vi "Tester.vi"() -> ()   [LabVIEW 2015]
uses:
  controls/Treatment Parameters.ctl
  controls/Results.ctl
panel:
  out "adjust limbus time":u32
  out "sclera plane time":u32
  in  "Results folder":path=path "S:/Dropbox/clients/BELKIN/Results Small"
  in  "Treatment":T1={"Location"=25.0, "Width"=10.0, "Search"=enum."Lower"}
  out "error out":errorcluster
  in  "Image folder":path=path "S:/Dropbox/clients/BELKIN/Images and Requirements/BELKIN_-_Basler-2015-10-05/BELKIN - Basler/Representative Subset"
  out "Output Image":T2(plugin-control)
  out "Input Image":T2(plugin-control)
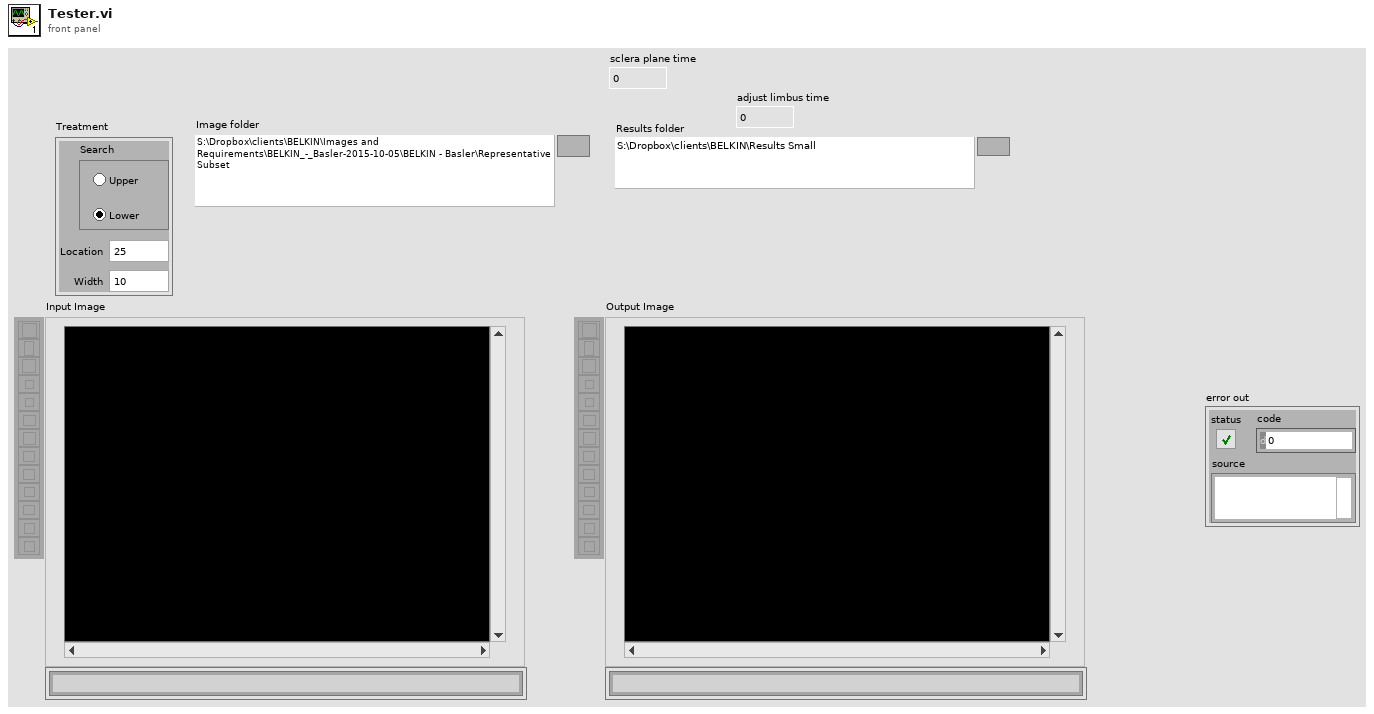
[diagram p1: front panel]
types:
  T1 = typedef "Treatment Parameters.ctl" = cluster{"Location":dbl, "Width":dbl, "Search":enum32{"Upper", "Lower"}}
  T2 = typedef "IMAQ Image.ctl" = refnum<image>
  T3 = typedef "Results.ctl" = cluster{"Center X":i32, "Center Y":i32, "Radius X":i32, "Radius Y":i32, "Circle Match Score":i32, "Sclera Score":dbl, "Circle Fit Strength":i32, "Circle Match Threshold":i32}
  T4 = typedef "Images.ctl" = cluster{"Input":T2, "Output":T2, "BufferGray1":T2, "BufferGray2":T2, "TemplatesDown":T2[], "TemplatesUp":T2[], "BufferColor1":T2, "GreenPlane":T2, "ScleraPlane":T2, "RedPlane":T2, "BluePlane":T2}
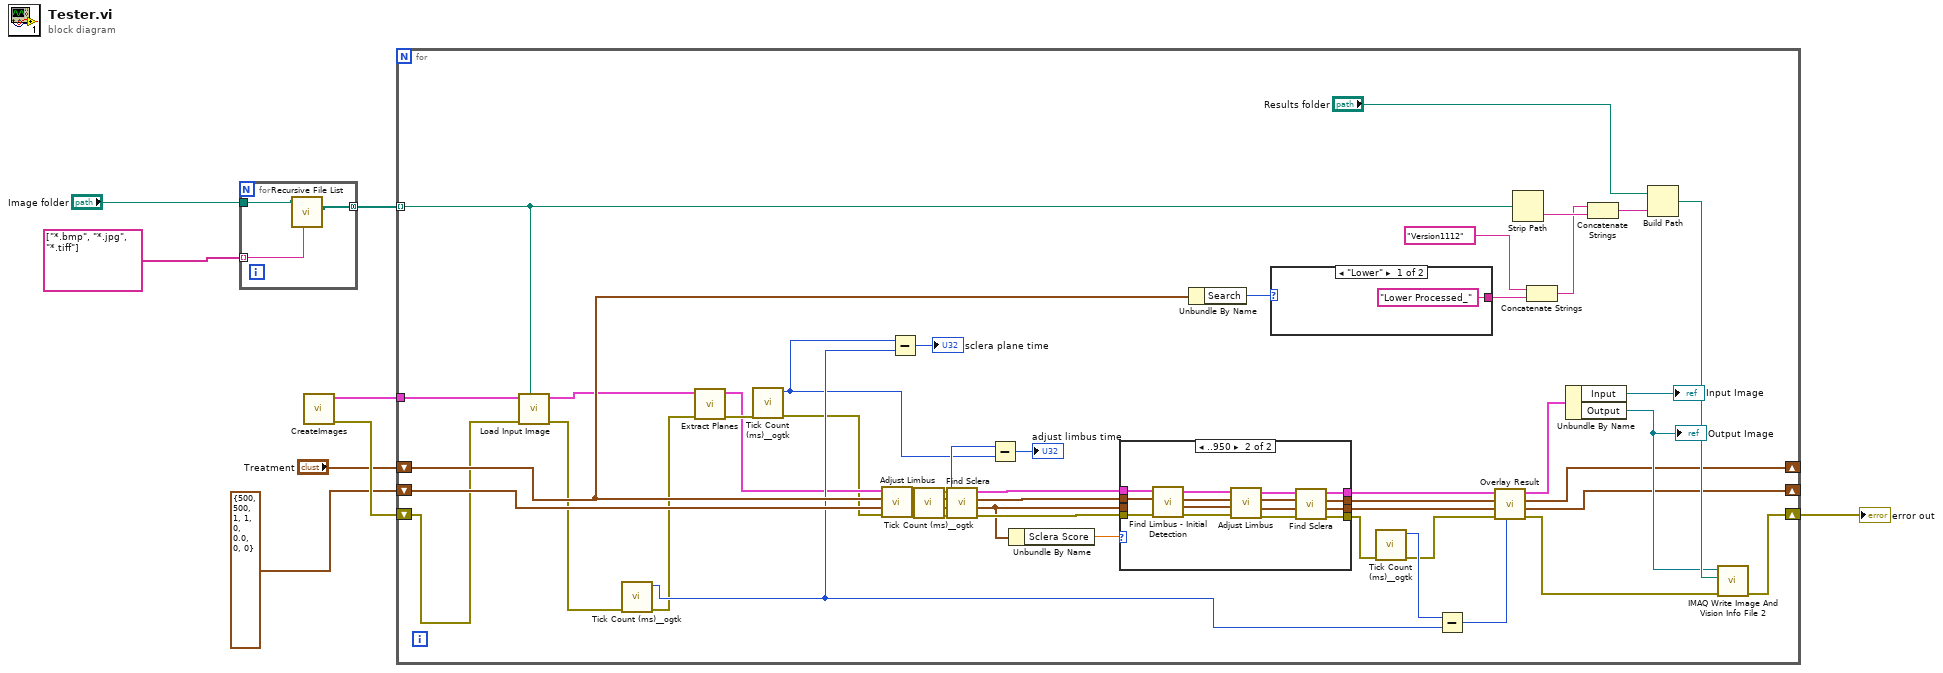
[diagram p0: block diagram]
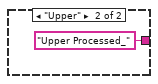
[diagram p3: hidden frame]
diagram:
  n1 = for {
    tunnel: "Image folder" -> [w11]
    tunnel: [w10] -> w7 mode=concatenating
    tunnel: string[] ["*.bmp", "*.jpg", "*.tiff"] -> [w9] mode=indexing
    n2 = call <vilib>:"Recursive File List.vi"("pattern"=w9, "Folder Path"=w11) -> ("All Files in Dir"=w10:path[])  [unwired: 5 in, 4 out]
  }
  n3 = call "CreateImages.vi"() -> ("error out"=w4:errorcluster, "Images"=w5:T4)  [unwired: 10 in]
  n4 = for {
    tunnel: w7 -> [w49] mode=indexing
    tunnel: w5 -> [w48]
    shift-right: [w54] -> w3
    shift-left: w4 -> [w24]
    shift-right: [w28] -> _
    shift-left: "Treatment" -> [w30]
    shift-right: [w27] -> _
    shift-left: T3 {"Center X"=500, "Center Y"=500, "Radius X"=1, "Radius Y"=1, "Circle Match Score"=0, "Sclera Score"=0.0, "Circle Fit Strength"=0, "Circle Match Threshold"=0} ("Results Out") -> [w29]
    n5 = call "Load Input Image.vi"("Path"=w49, "error in (no error)"=w24, "Images"=w48) -> ("error out"=w23:errorcluster, "Images"=w15:T4)  [unwired: 7 in]
    n6 = call <userlib>:"Tick Count (ms)__ogtk.vi"("error in (no error)"=w23) -> ("error out"=w16:errorcluster, "millisecond timer value"=w21:u32)  [unwired: 9 in]
    n7 = call "Extract Planes.vi"("error in (no error)"=w16, "Images"=w15) -> ("error out"=w17:errorcluster, "Images"=w14:T4)  [unwired: 8 in]
    n8 = call <userlib>:"Tick Count (ms)__ogtk.vi"("error in (no error)"=w17) -> ("error out"=w13:errorcluster, "millisecond timer value"=w12:u32)  [unwired: 9 in]
    n9 = call "Adjust Limbus.vi"("error in (no error)"=w13, "Results"=w29, "Treatment"=w30, "Images"=w14) -> ("error out"=w35:errorcluster, "Results"=w37:T3, "Treatment"=w36:T1, "Images"=w34:T4)  [unwired: 4 in]
    n10 = Subtract(x=w12, y=w21) -> (x-y=→"sclera plane time":u32)
    n11 = call <userlib>:"Tick Count (ms)__ogtk.vi"("error in (no error)"=w35) -> ("error out"=w22:errorcluster, "millisecond timer value"=w18:u32)  [unwired: 9 in]
    n12 = call "Find Sclera.vi"("error in (no error)"=w22, "Results"=w37, "Treatment"=w36, "Images"=w34) -> ("error out"=w31:errorcluster, "Results"=w25:T3, "Treatment"=w32:T1, "Images"=w33:T4)  [unwired: 4 in]
    n13 = Subtract(x=w18, y=w12) -> (x-y=→"adjust limbus time":u32)
    n14 = Unbundle By Name(w25) -> ("Sclera Score"=w26:dbl)
    n15 = case shown="..950" w26 {
      tunnel: [w63 w78] -> w52
      tunnel: [w62 w77] -> w51
      tunnel: [w61 w76] -> w50
      tunnel: [w60 w68] -> w42
      tunnel: w33 -> [w63 w66]
      tunnel: w32 -> [w62 w65]
      tunnel: w31 -> [w60 w64]
      tunnel: w25 -> [w61 _]
      frame 951.. {
      }
      frame ..950 {
        n16 = call "Find Limbus - Initial Detection.vi"("error in (no error)"=w64, "Treatment in"=w65, "Images in"=w66) -> ("error out"=w67:errorcluster, "Results"=w71:T3, "Treatment Out"=w72:T1, "Images out"=w75:T4)  [unwired: 5 in]
        n17 = call "Adjust Limbus.vi"("error in (no error)"=w67, "Results"=w71, "Treatment"=w72, "Images"=w75) -> ("error out"=w73:errorcluster, "Results"=w69:T3, "Treatment"=w70:T1, "Images"=w74:T4)  [unwired: 4 in]
        n18 = call "Find Sclera.vi"("error in (no error)"=w73, "Results"=w69, "Treatment"=w70, "Images"=w74) -> ("error out"=w68:errorcluster, "Results"=w76:T3, "Treatment"=w77:T1, "Images"=w78:T4)  [unwired: 4 in]
      }
    }
    n19 = Unbundle By Name(w30) -> ("Search"=w53:enum32{"Upper", "Lower"})
    n20 = case shown="\"Lower\"" w53 {
      tunnel: ["Lower Processed_" ("string") "Upper Processed_" ("string")] -> w58
      frame "Lower" {
      }
      frame "Upper" {
      }
    }
    n21 = call <userlib>:"Tick Count (ms)__ogtk.vi"("error in (no error)"=w42) -> ("error out"=w40:errorcluster, "millisecond timer value"=w41:u32)  [unwired: 9 in]
    n22 = Subtract(x=w41, y=w21) -> (x-y=w38:u32)
    n23 = call "Overlay Result.vi"("Processing Time"=w38, "error in (no error)"=w40, "Results"=w50, "Treatment"=w51, "Images"=w52) -> ("error out"=w39:errorcluster, "Results Out"=w27:T3, "Treatment Out"=w28:T1, "Images"=w47:T4)  [unwired: 3 in]
    n24 = Strip Path(path=w49) -> (name=w59:string)  [unwired: 1 out]
    n25 = Concatenate Strings("Version1112" ("string"), w58) -> (w44:string)
    n26 = Unbundle By Name(w47) -> ("Input"=→"Input Image":T2, "Output"=w46:T2)
    "Output Image" <- w46
    n27 = Concatenate Strings(w44, w59) -> (w57:string)
    n28 = Build Path(base path="Results folder", name or relative path=w57) -> (appended path=w55:path)
    n29 = call "IMAQ Write Image And Vision Info File 2"("error in (no error)"=w39, "File Path"=w55, "Image"=w46) -> ("error out"=w54:errorcluster)  [unwired: 7 in, 1 out]
  }
  "error out" <- w3
